vi "RUSHVision.vi"(7 "Enable Vision":bool, 8 "Mask Image":T5, 9 "Orig Image":T5, 10 "Camera Settings":T4, 11 "CameraDevRef":T6) -> (2 "Aspect Ratio":dbl[](array[numeric]), 3 "Target Info":T8(array[cluster]))   [LabVIEW 2011]
uses:
  <vilib>/Rock Robotics/WPI/Camera/WPI_CameraDevRef.ctl
  <vilib>/vision/Image Controls.llb/IMAQ Image.ctl
  <vilib>/Rock Robotics/WPI/Camera/WPI_CameraImageSize.ctl
  <vilib>/Rock Robotics/WPI/Camera/WPI_CameraWhite Balance Values.ctl
  <vilib>/Rock Robotics/WPI/Camera/WPI_CameraExposure Values.ctl
  <vilib>/vision/NI_Vision_Development_Module.lvlib
panel:
  in  "View 2":bool
  in  "Processing":enum32{"Color", "Intensity", "Intensity Open"}(tab)=enum."Intensity"
  in  "Luminance":i32=255
  in  "Saturation":i32=255
  in  "Hue":i32(knob)=65 scale=0.0..255.0
  in  "Margins":cluster{"Hue":i32, "Sat":i32, "Lum":i32}={"Hue"=20, "Sat"=27, "Lum"=30} {"Sat" scale=0.0..40.0; "Lum" scale=0.0..40.0; "Hue" scale=0.0..40.0}
  in  "Range":cluster{"Lower value":sgl, "Upper value":sgl}={"Lower value"=153.36957, "Upper value"=255.0} {"Lower value" scale=0.0..255.0; "Upper value" scale=0.0..255.0}
  in  "Range 2":cluster{"Lower value":sgl, "Upper value":sgl}={"Lower value"=123.804344, "Upper value"=255.0} {"Lower value" scale=0.0..255.0; "Upper value" scale=0.0..255.0}
  in  "Particle Count Limit":i32=8
  in  "Area Size Limit":i32=444
  in  "Score Limits":T7={"Rect Coverage"=76.0, "Aspect Ratio"=40.0, "X Edge Strength"=40.0, "Y Edge Strength"=60.0}
  in  "View":bool
  out "Original Image":T5(plugin-control)
  out "Processed Image":T5(plugin-control)
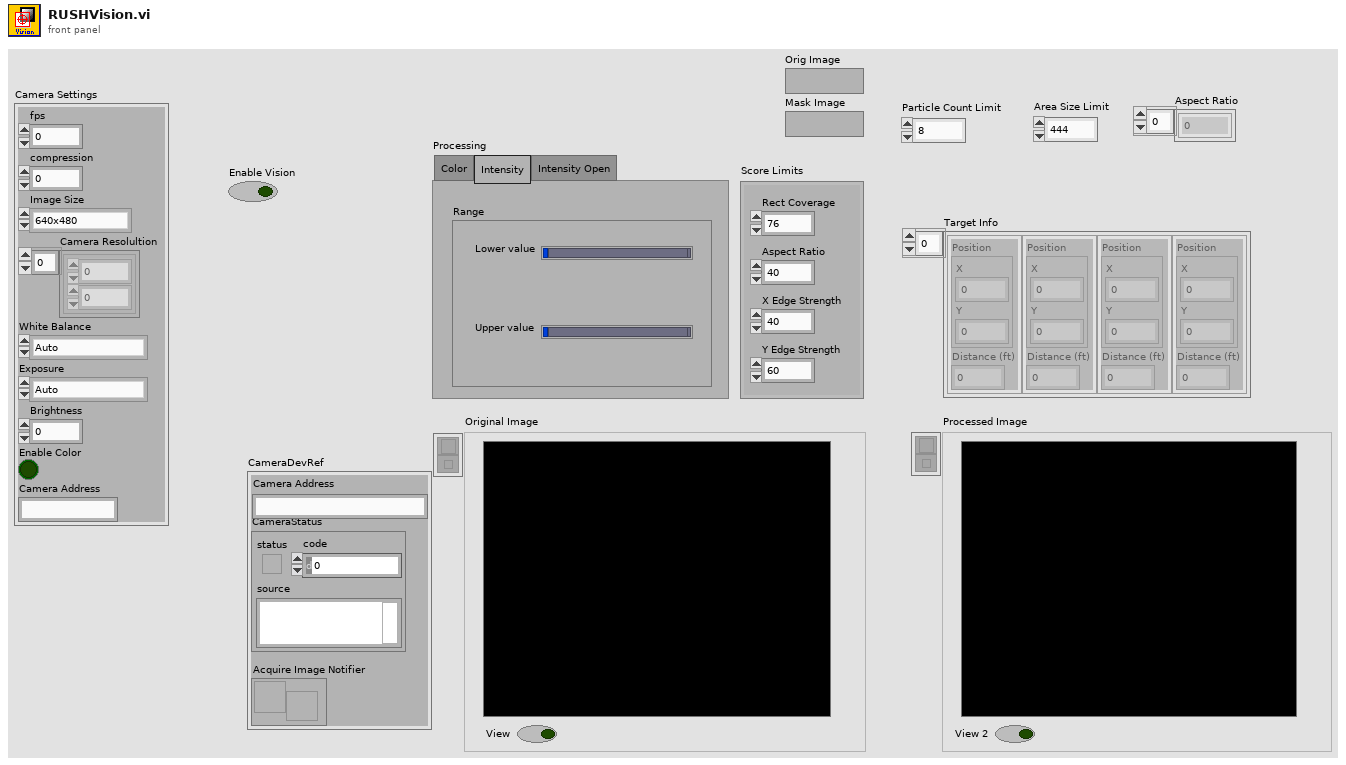
[diagram p1: front panel]
types:
  T1 = typedef "WPI_CameraImageSize.ctl" = enum16{"640x480", "320x240", "160x120"}
  T2 = typedef "WPI_CameraWhite Balance Values.ctl" = enum16{"Auto", "Fixed indoor", "Fixed outdoor 1", "Fixed outdoor 2", "Fixed fluorescent 1", "Fixed fluorescent 2", "Hold current"}
  T3 = typedef "WPI_CameraExposure Values.ctl" = enum16{"Auto", "Flicker-free 50 Hz", "Flicker-free 60 Hz", "Hold current"}
  T4 = cluster{"fps":i32, "compression":i32, "Image Size":T1, "Camera Resolultion":cluster{i32, i32}[], "White Balance":T2, "Exposure":T3, "Brightness":dbl, "Enable Color":bool, "Camera Address":string}
  T5 = typedef "IMAQ Image.ctl" = refnum<image>
  T6 = typedef "WPI_CameraDevRef.ctl" = cluster{"Camera Address":string, "CameraStatus":errorcluster, "Acquire Image Notifier":refnum<notifier>}
  T7 = cluster{"Rect Coverage":dbl, "Aspect Ratio":dbl, "X Edge Strength":dbl, "Y Edge Strength":dbl}
  T8 = cluster{"Position":cluster{"X":dbl, "Y":dbl}, "Distance (ft)":dbl}[]
  T9 = enum32{"AutoM", "Close", "Dilate", "Erode", "Gradient", "Gradient out", "Gradient in", "Hit miss", "Open", "PClose", "POpen", "Thick", "Thin"}
  T10 = cluster{cluster{"Left":dbl, "Top":dbl, "Right":dbl, "Bottom":dbl}, dbl[]}[]
  T11 = cluster{"Left":dbl, "Top":dbl, "Right":dbl, "Bottom":dbl}
  T12 = cluster{"Target Center (-1 to 1)":cluster{"X":dbl, "Y":dbl}, "Distance (ft)":dbl}
  T13 = cluster{"Target Center (-1 to 1)":cluster{"X":dbl, "Y":dbl}, "Distance (ft)":dbl}[]
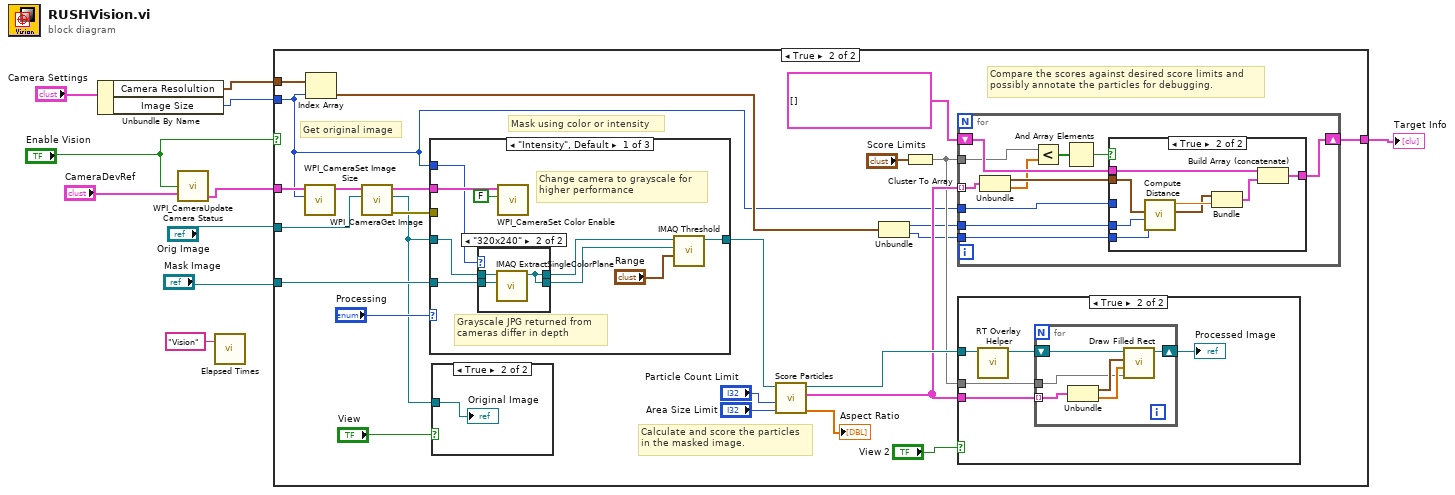
[diagram p0: block diagram]
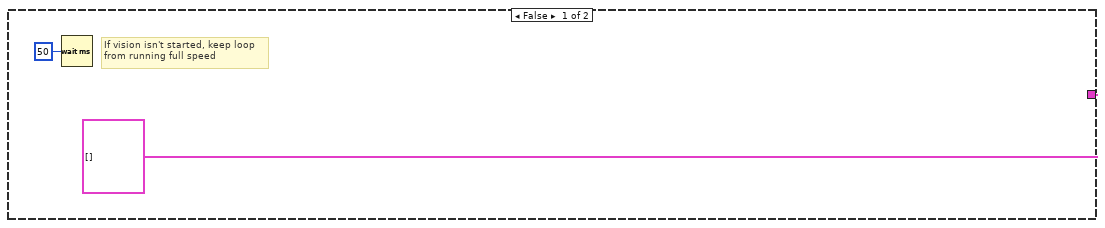
[diagram p2: hidden frame]
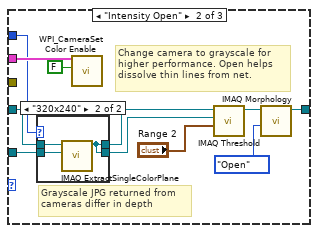
[diagram p4: hidden frame]
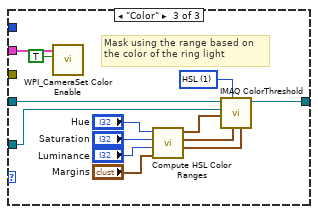
[diagram p6: hidden frame]
diagram:
  n1 = Unbundle By Name("Camera Settings") -> ("Camera Resolultion"=w1:cluster{i32, i32}[], "Image Size"=w2:T1)
  n2 = call <vilib>:"WPI_CameraUpdate Camera Status.vi"("CameraDevRef In"="CameraDevRef", "Enable Vision"="Enable Vision") -> ("CameraDevRef Out"=w9:T6)  [unwired: 3 in]
  n3 = call "Elapsed Times.vi"("Call Name"="Vision") -> ()  [unwired: 2 in, 1 out]
  n4 = case shown="True" "Enable Vision" {
    tunnel: "Orig Image" -> [_ w28]
    tunnel: w9 -> [_ w24]
    tunnel: "Mask Image" -> [_ w17]
    tunnel: w1 -> [_ w21]
    tunnel: w2 -> [_ w15]
    tunnel: [T8 [] w13] -> w5
    frame False {
      # "If vision isn't started, keep loop\nfrom running full speed"
      n5 = Wait (ms)(milliseconds to wait=u32 50) -> ()  [unwired: 1 out]
    }
    frame True {
      # "Compare the scores against desired score limits and\npossibly annotate the particles for debugging."
      # "Calculate and score the particles\nin the masked image."
      # "Mask using color or intensity"
      # "Get original image"
      n6 = call <vilib>:"WPI_CameraSet Image Size.vi"("Image Size"=w15, "CameraDevRef"=w24) -> ("CameraDevRef Out"=w25:T6)  [unwired: 8 in, 1 out]
      n7 = Index Array(array=w21, index=w15) -> (element=w18:cluster{i32, i32})
      n8 = call <vilib>:"WPI_CameraGet Image.vi"("Image"=w28, "CameraDevRef"=w25) -> ("error out"=w26:errorcluster, "Image Out"=w16:T5, "CameraDevRef Out"=w27:T6)  [unwired: 7 in]
      n9 = case shown="\"Intensity\", Default" "Processing" {
        tunnel: w16 -> [w42 w54 w80]
        tunnel: [w45 w59 w79] -> w22
        tunnel: w27 -> [w43 w57 w70]
        tunnel: w26 -> [_ _ _]
        tunnel: w17 -> [w41 w55 w68]
        tunnel: w15 -> [w40 w56 _]
        frame "Intensity", Default {
          # "Grayscale JPG returned from\ncameras differ in depth"
          # "Change camera to grayscale for\nhigher performance"
          n10 = case shown="\"320x240\"" w40 {
            tunnel: w42 -> [w48 w51]
            tunnel: w41 -> [w47 w50]
            tunnel: [w48 w49] -> w39
            tunnel: [w47 w49] -> w38
            frame "640x480", Default {
            }
            frame "320x240" {
              n11 = call "IMAQ ExtractSingleColorPlane"("Image Dst"=w50, "Image Src"=w51) -> ("Image Dst Out"=w49:T5)  [unwired: 8 in, 1 out]
            }
          }
          n12 = call <vilib>:"WPI_CameraSet Color Enable.vi"("Color Enabled"=FALSE, "CameraDevRef"=w43) -> ()  [unwired: 8 in, 2 out]
          n13 = call "IMAQ Threshold"("Range"="Range", "Image Dst"=w38, "Image Src"=w39) -> ("Image Dst Out"=w45:T5)  [unwired: 3 in, 5 out]
        }
        frame "Intensity Open" {
          # "Grayscale JPG returned from\ncameras differ in depth"
          # "Change camera to grayscale for\nhigher performance. Open helps\ndissolve thin lines from net."
          n14 = case shown="\"320x240\"" w56 {
            tunnel: w54 -> [w64 w67]
            tunnel: w55 -> [w63 w66]
            tunnel: [w64 w65] -> w53
            tunnel: [w63 w65] -> w52
            frame "640x480", Default {
            }
            frame "320x240" {
              n15 = call "IMAQ ExtractSingleColorPlane"("Image Dst"=w66, "Image Src"=w67) -> ("Image Dst Out"=w65:T5)  [unwired: 8 in, 1 out]
            }
          }
          n16 = call <vilib>:"WPI_CameraSet Color Enable.vi"("Color Enabled"=FALSE, "CameraDevRef"=w57) -> ()  [unwired: 8 in, 2 out]
          n17 = call "IMAQ Threshold"("Range"="Range 2", "Image Dst"=w52, "Image Src"=w53) -> ("Image Dst Out"=w60:T5)  [unwired: 3 in, 5 out]
          n18 = call "IMAQ Morphology"("Operation"=T9."Open", "Image Src"=w60) -> ("Image Dst Out"=w59:T5)  [unwired: 8 in, 1 out]
        }
        frame "Color" {
          w78 = u16 1 items=["RGB", "HSL", "HSV", "HSI"] ("Color Mode")
          # "Mask using the range based on\nthe color of the ring light"
          n19 = call <vilib>:"WPI_CameraSet Color Enable.vi"("Color Enabled"=TRUE, "CameraDevRef"=w70) -> ()  [unwired: 8 in, 2 out]
          n20 = call "Compute HSL Color Ranges.vi"("Margins"="Margins", "Luminance"="Luminance", "Saturation"="Saturation", "Hue"="Hue") -> ("Lum Range"=w75:cluster{i32, i32}, "Sat Range"=w76:cluster{i32, i32}, "Hue Range"=w77:cluster{i32, i32})  [unwired: 5 in]
          n21 = call "IMAQ ColorThreshold"("Blue or Luma or Val or Inten Range"=w75, "Green or Sat Range"=w76, "Color Mode"=w78, "Red or Hue Range"=w77, "Image Dst"=w68, "Image Src"=w80) -> ("Image Dst Out"=w79:T5)  [unwired: 4 in, 1 out]
        }
      }
      n22 = case shown="True" "View" {
        tunnel: w16 -> [_ w92]
        frame False {
        }
        frame True {
          "Original Image" <- w92
        }
      }
      n23 = call "Score Particles.vi"("Area Size Limit"="Area Size Limit", "Particle Count Limit"="Particle Count Limit", "Image Refnum in"=w22) -> ("Aspect Ratio"=→"Aspect Ratio":dbl[], "Scored Particle Info"=w33:T10, "Image Refnum out"=w36:T5)  [unwired: 6 in]
      n24 = Unbundle(w18) -> (w20:i32, w19:i32)
      n25 = Cluster To Array(cluster="Score Limits") -> (array=w31:dbl[])
      n26 = for {
        shift-right: [w102] -> w13
        shift-left: T8 [] -> [w103]
        tunnel: w20 -> [w101]
        tunnel: w33 -> [w99] mode=indexing
        tunnel: w31 -> [w94]
        tunnel: w15 -> [w98]
        tunnel: w19 -> [w93]
        n27 = Unbundle(w99) -> (w100:T11, w95:dbl[])
        n28 = Less?(x=w94, y=w95) -> (x < y?=w97:bool[])
        n29 = And Array Elements(Boolean array=w97) -> (logical AND=w96:bool)
        n30 = case shown="True" w96 {
          tunnel: w103 -> [w104 w112]
          tunnel: [w104 w111] -> w102
          tunnel: w100 -> [_ w107]
          tunnel: w101 -> [_ w109]
          tunnel: w98 -> [_ _]
          tunnel: w93 -> [_ w106]
          frame False {
          }
          frame True {
            n31 = call "Compute Distance.vi"("Y Image Resolution"=w106, "X Image Resolution"=w109, "Bounding Box"=w107) -> ("Target Center (-1 to 1)"=w105:cluster{"X":dbl, "Y":dbl}, "Distance (ft)"=w108:dbl)  [unwired: 7 in]
            n32 = Bundle("Target Center (-1 to 1)"=w105, "Distance (ft)"=w108) -> (w110:T12)  [unwired: 1 in]
            n33 = Build Array (concatenate)(w112, w110) -> (w111:T13)
          }
        }
      }
      n34 = case shown="True" "View 2" {
        tunnel: w36 -> [_ w82]
        tunnel: w33 -> [_ w84]
        tunnel: w31 -> [_ w83]
        frame False {
        }
        frame True {
          n35 = call "RT Overlay Helper.vi"("Refnum in"=w82) -> ("Refnum out"=w85:T5)  [unwired: 10 in]
          n36 = for {
            shift-right: [w90] -> w81
            shift-left: w85 -> [w91]
            tunnel: w84 -> [w87] mode=indexing
            tunnel: w83 -> [w86]
            n37 = Unbundle(w87) -> (w88:T11, w89:dbl[])
            n38 = call "Draw Filled Rect.vi"("Limits"=w86, "Scores"=w89, "Bounding Box"=w88, "image in"=w91) -> ("image out"=w90:T5)  [unwired: 7 in]
          }
          "Processed Image" <- w81
        }
      }
    }
  }
  "Target Info" <- w5
